vi "checkIfAxesAreHomed.vi"(8 "error in (no error)":errorcluster, 9 "check these axes homed":T1[](array[typedef]), 11 "sub-systems in":refnum<class "sub-systems.lvclass">) -> (0 "error out":errorcluster, 1 "Homed=T":bool, 3 "sub-systems out":refnum<class "sub-systems.lvclass">)   [LabVIEW 2019, in "sub-systems.lvclass"]
uses:
  sub-systems.lvclass
  APARMainSubvis/VXM Public API/mmWaveAxis.ctl
  sub-systems.lvclass/sub-systems.ctl
  VSMx2/VXMx2.lvclass
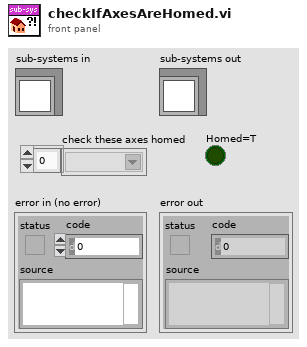
[diagram p1: front panel]
types:
  T1 = typedef "mmWaveAxis.ctl" = string
  T2 = typedef "Velmex VXM.lvlib/VXM Axis.ctl" = u16
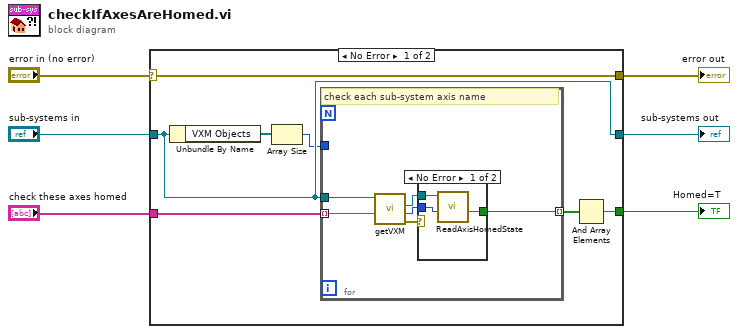
[diagram p0: block diagram]
diagram:
  n1 = case shown="No Error" "error in (no error)" {
    selector: "error in (no error)" -> [w13 w24]
    tunnel: [w13 w24] -> w5
    tunnel: [w11 w23] -> w3
    tunnel: "sub-systems in" -> [w11 w23]
    tunnel: "check these axes homed" -> [w12 _]
    tunnel: [w7 _] -> w1
    frame No Error {
      n2 = Unbundle By Name(w11) -> ("VXM Objects"=w10:refnum<class "VXMx2.lvclass">[])
      n3 = Array Size(array=w10) -> (size(s)=w9:i32)
      n4 = for {
        tunnel: w12 -> [w19] mode=indexing
        tunnel: w11 -> [w18]
        tunnel: w9 -> [_]
        tunnel: [w17] -> w8 mode=indexing
        # "check each sub-system axis name"
        n5 = call "getVXM.vi"("mmWave Axis Name"=w19, "sub-systems in"=w18) -> ("error out"=w16:errorcluster, "Axis (1..4)"=w15:T2, "VXMx2 out"=w14:refnum<class "VXMx2.lvclass">)  [unwired: 5 in, 2 out]
        n6 = case shown="No Error" w16 {
          tunnel: w15 -> [w22 _]
          tunnel: w14 -> [w21 _]
          tunnel: [w20 _] -> w17
          frame No Error {
            n7 = call "ReadAxisHomedState.vi"("Axis (1..4)"=w22, "VXMx2 in"=w21) -> ("Homed=T"=w20:bool)  [unwired: 7 in, 2 out]
          }
          frame Error {
          }
        }
      }
      n8 = And Array Elements(Boolean array=w8) -> (logical AND=w7:bool)
    }
    frame Error {
    }
  }
  "error out" <- w5
  "sub-systems out" <- w3
  "Homed=T" <- w1
